vi "Read Serial Configs.vi"(8 "error in (no error)":errorcluster, 10 "Item Ref in":T2 format="%.0x", 11 "Refnum in":T1) -> (0 "error out":errorcluster, 2 "Item Ref out":T2 format="%.0x", 3 "Refnum out":T1)   [LabVIEW 2021, in "Modbus Master System Explorer.lvlib"]
uses:
  Modbus Master System Explorer.lvlib
  <vilib>/Utility/config.llb/Config Data RefNum.ctl
  <vilib>/NI VeriStand/Custom Device API/Custom Device Item Ref.ctl
  Shared/Controls/Flow Control.ctl
  Shared/Controls/Serial Type.ctl
  Shared/Controls/Parity.ctl
  <vilib>/Utility/config.llb/Read Key (String).vi
  <vilib>/Utility/config.llb/Read Key (U32).vi
  <vilib>/Utility/config.llb/NI_LVConfig.lvlib
  Shared/Modbus Master Shared.lvlib
  <vilib>/NI VeriStand/Custom Device API/Custom Device API.lvlib
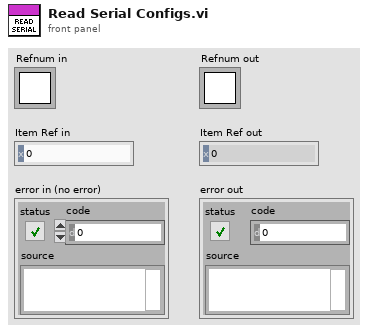
[diagram p1: front panel]
types:
  T1 = typedef "NI_LVConfig.lvlib/Config Data RefNum.ctl" = refnum<k1>
  T2 = typedef "Custom Device API.lvlib/Custom Device Item Ref.ctl" = u64
  T3 = typedef "Modbus Master Shared.lvlib/Parity.ctl" = u16
  T4 = typedef "Modbus Master Shared.lvlib/Serial Type.ctl" = enum16{"RTU", "ASCII"}
  T5 = typedef "Modbus Master Shared.lvlib/Flow Control.ctl" = u16
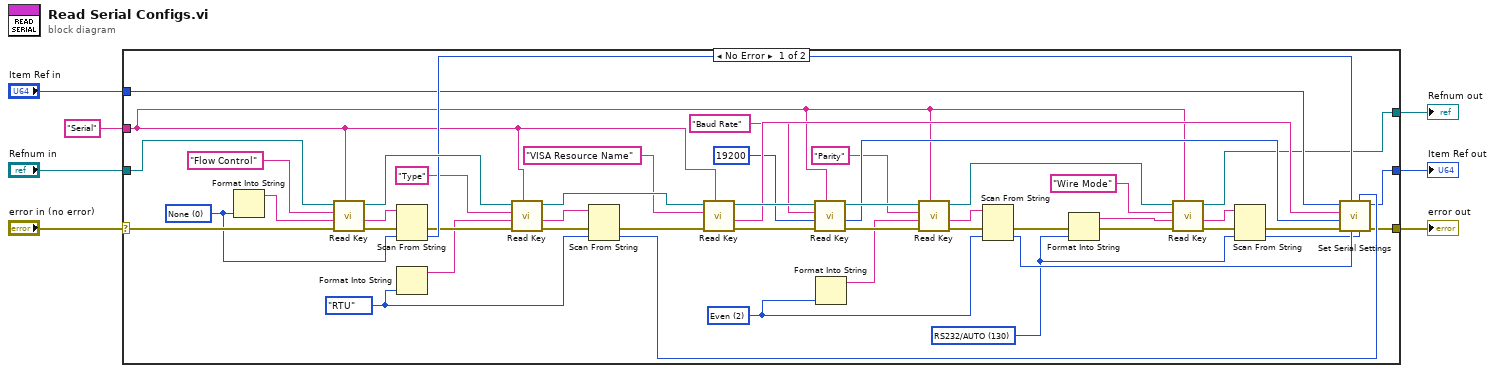
[diagram p0: block diagram]
diagram:
  n1 = case shown="No Error" "error in (no error)" {
    selector: "error in (no error)" -> [w50 w57]
    tunnel: "Refnum in" -> [w55 w56]
    tunnel: "Serial" ("section") -> [w17 _]
    tunnel: [w29 w57] -> w4
    tunnel: [w28 w58] -> w3
    tunnel: "Item Ref in" -> [w27 w58]
    tunnel: [w18 w56] -> w1
    frame No Error {
      w15 = i16 130 items=["Unknown"=-1, "RS485/Wire4"=0, "RS485/Wire2-EchoDTR"=1, "RS485/Wire2-CtrlDTR"=2, "RS485/Wire2-Auto"=3, "RS232/DTE"=128, "RS232/DCE"=129, "RS232/AUTO"=130] ("Serial Settings:Wire Mode")
      w22 = T3 2 items=["None", "Odd", "Even", "Mark", "Space"] ("parity (even)")
      w24 = Serial_Type."RTU" ("serial type")
      w26 = T5 0 items=["None", "XON/XOFF", "RTS/CTS", "XON/XOFF & RTS/CTS", "DTR/DSR", "XON/XOFF & DTR/DSR"] ("flow control (none)")
      n2 = Format Into String(w26) -> (resulting string=w25:string)  [unwired: 3 in, 1 out]
      n3 = call-poly <vilib>:"Read Key.vi"("section"=w17, "error in (no error)"=w50, "default value"=w25, "key"="Flow Control", "refnum"=w55) -> ("error out"=w44:errorcluster, "value"=w46:string, "refnum out"=w51:T1)  [unwired: 3 in, 1 out]
      n4 = Scan From String(input string=w46, error in=w44, default 1=w26) -> (error out=w43:errorcluster, output 1=w45:T5)  [unwired: 2 in, 2 out]
      n5 = Format Into String(w24) -> (resulting string=w23:string)  [unwired: 3 in, 1 out]
      n6 = call-poly <vilib>:"Read Key.vi"("section"=w17, "error in (no error)"=w43, "default value"=w23, "key"="Type", "refnum"=w51) -> ("error out"=w39:errorcluster, "value"=w42:string, "refnum out"=w54:T1)  [unwired: 3 in, 1 out]
      n7 = Scan From String(input string=w42, error in=w39, default 1=w24) -> (error out=w38:errorcluster, output 1=w40:T4)  [unwired: 2 in, 2 out]
      n8 = call-poly <vilib>:"Read Key.vi"("section"=w17, "error in (no error)"=w38, "key"="VISA Resource Name", "refnum"=w54) -> ("error out"=w49:errorcluster, "value"=w36:string, "refnum out"=w53:T1)  [unwired: 4 in, 1 out]
      n9 = call-poly <vilib>:"Read Key.vi"("section"=w17, "error in (no error)"=w49, "default value"=u32 19200, "key"="Baud Rate", "refnum"=w53) -> ("error out"=w48:errorcluster, "value"=w34:u32, "refnum out"=w52:T1)  [unwired: 3 in, 1 out]
      n10 = Format Into String(w22) -> (resulting string=w21:string)  [unwired: 3 in, 1 out]
      n11 = call-poly <vilib>:"Read Key.vi"("section"=w17, "error in (no error)"=w48, "default value"=w21, "key"="Parity", "refnum"=w52) -> ("error out"=w30:errorcluster, "value"=w32:string, "refnum out"=w19:T1)  [unwired: 3 in, 1 out]
      n12 = Scan From String(input string=w32, error in=w30, default 1=w22) -> (error out=w11:errorcluster, output 1=w31:T3)  [unwired: 2 in, 2 out]
      n13 = Format Into String(error in=w11, w15) -> (resulting string=w16:string, error out=w10:errorcluster)  [unwired: 2 in]
      n14 = call-poly <vilib>:"Read Key.vi"("section"=w17, "error in (no error)"=w10, "default value"=w16, "key"="Wire Mode", "refnum"=w19) -> ("error out"=w9:errorcluster, "value"=w20:string, "refnum out"=w18:T1)  [unwired: 3 in, 1 out]
      n15 = Scan From String(input string=w20, error in=w9, default 1=w15) -> (error out=w8:errorcluster, output 1=w14:i16)  [unwired: 2 in, 2 out]
      n16 = call "Set Serial Settings.vi"("Wire Mode"=w14, "serial type"=w40, "parity (even)"=w31, "flow control (none)"=w45, "error in (no error)"=w8, "baud rate"=w34, "VISA resource name"=w36, "Item Ref in"=w27) -> ("error out"=w29:errorcluster, "Item Ref out"=w28:T2)  [unwired: 2 in]
    }
    frame Error {
    }
  }
  "error out" <- w4
  "Item Ref out" <- w3
  "Refnum out" <- w1
